vi "ReadErrorInfo.vi"(8 "error in (no error)":errorcluster, 11 "object in":refnum<class "Reply Message.lvclass">) -> (0 "error out":errorcluster, 2 "Error info":T1, 3 "object out":refnum<class "Reply Message.lvclass">)   [LabVIEW 2018, in "ClientMessaging.lvlib" / "Reply Message.lvclass"]
uses:
  Reply Message.lvclass
  Reply Message.lvclass/Reply Message.ctl
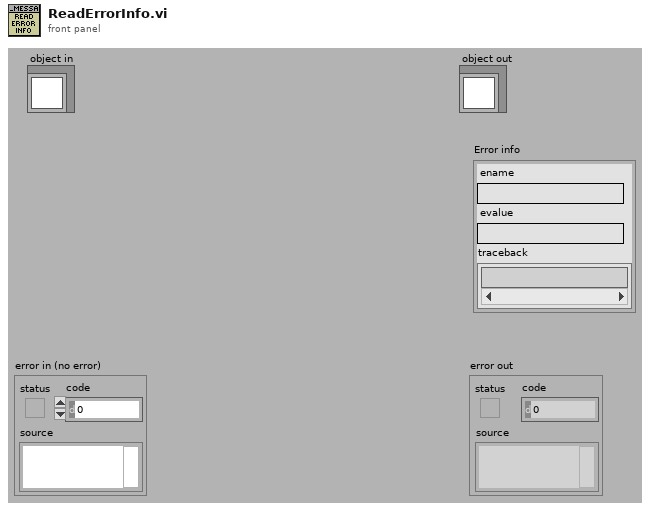
[diagram p1: front panel]
types:
  T1 = cluster{"ename":string, "evalue":string, "traceback":string[]}
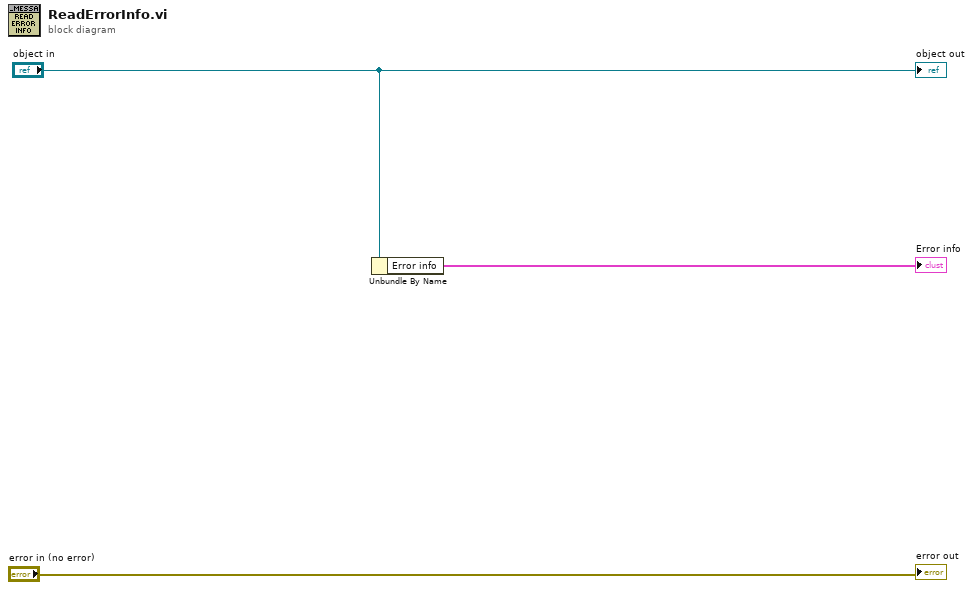
[diagram p0: block diagram]
diagram:
  n1 = Unbundle By Name("object in") -> ("Error info"=→"Error info":T1)
  "error out" <- "error in (no error)"
  "object out" <- "object in"
